vi "TCP Client.vi"() -> ()   [LabVIEW 2014]
panel:
  in  "주소":string
  in  "x .or. y?":bool
  out "웨이브폼 그래프":dbl[](graph)
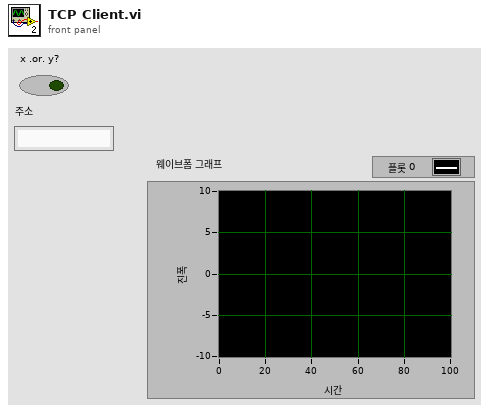
[diagram p1: front panel]
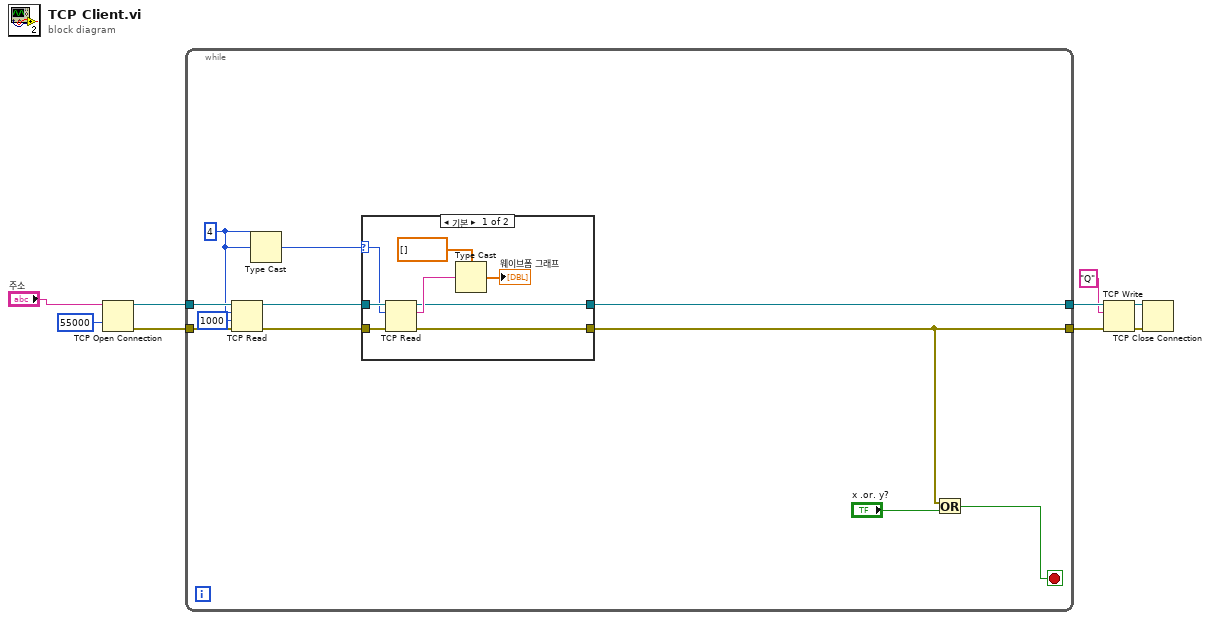
[diagram p0: block diagram]
diagram:
  n1 = TCP Open Connection(address="주소", remote port or service name=u16 55000 ("원격 포트 또는 서비스 이름")) -> (connection ID=w8:refnum<k5>, error out=w7:errorcluster)  [unwired: 3 in]
  n2 = while {
    tunnel: w8 -> [w19]
    tunnel: w7 -> [w20]
    tunnel: [w13] -> w5
    tunnel: [w10] -> w6
    stop <- w12 stop-if-true
    w16 = 4
    n3 = TCP Read(connection ID=w19, bytes to read=w16, error in (no error)=w20, 9:1000 ("타임아웃 ms (25000)")) -> (connection ID out=w15:refnum<k5>, error out=w14:errorcluster)  [unwired: 1 in, 1 out]
    n4 = Type Cast(type=w16, x=w16) -> (*(type *) &x=w17:i32)
    n5 = case shown="기본" w17 {
      selector: w17 -> [w26 _]
      tunnel: w15 -> [w28 w30]
      tunnel: w14 -> [w27 w29]
      tunnel: [w22 w30] -> w13
      tunnel: [w21 w29] -> w10
      frame Default {
        n6 = TCP Read(connection ID=w28, bytes to read=w26, error in (no error)=w27) -> (connection ID out=w22:refnum<k5>, data out=w25:string, error out=w21:errorcluster)  [unwired: 2 in]
        n7 = Type Cast(type=dbl[] [] ("웨이브폼 그래프"), x=w25) -> (*(type *) &x=→"웨이브폼 그래프":dbl[])
      }
      frame 0 {
      }
    }
    n8 = Or(x=w10, y="x .or. y?") -> (x .or. y?=w12:bool)
  }
  n9 = TCP Write(connection ID=w5, data in="Q" ("데이터 입력"), error in (no error)=w6) -> (connection ID out=w2:refnum<k5>, error out=w3:errorcluster)  [unwired: 1 in, 1 out]
  n10 = TCP Close Connection(connection ID=w2, error in (no error)=w3) -> ()  [unwired: 1 in, 2 out]
